vi "sv_Extract Indices from RPM Curve.vi"(2 "rpm segment":T1={"from [rpm]"=2000.0, "to [rpm]"=4000.0, "rpm increment [rpm]"=100.0} {"rpm increment [rpm]" min=1.0 format="%.2f"; "to [rpm]" format="%.2f"; "from [rpm]" format="%.2f"}, 3 "rpm vs. indices":cluster{"indices":dbl[], "speed [rpm]":dbl[]} {"speed [rpm]" format="%.2f"; "indices" format="%.2f"}) -> (0 "rpm0 and delta rpm [rpm]":cluster{"rpm0":dbl, "delta rpm":dbl} {"delta rpm" format="%.2f"; "rpm0" format="%.2f"}, 1 "indices":i32[](array[numeric]))   [LabVIEW 2017]
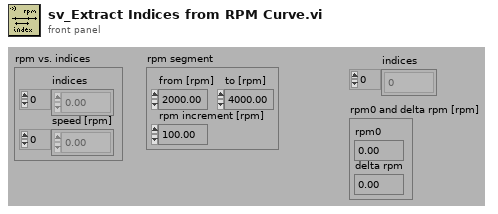
[diagram p1: front panel]
types:
  T1 = cluster{"from [rpm]":dbl, "to [rpm]":dbl, "rpm increment [rpm]":dbl}
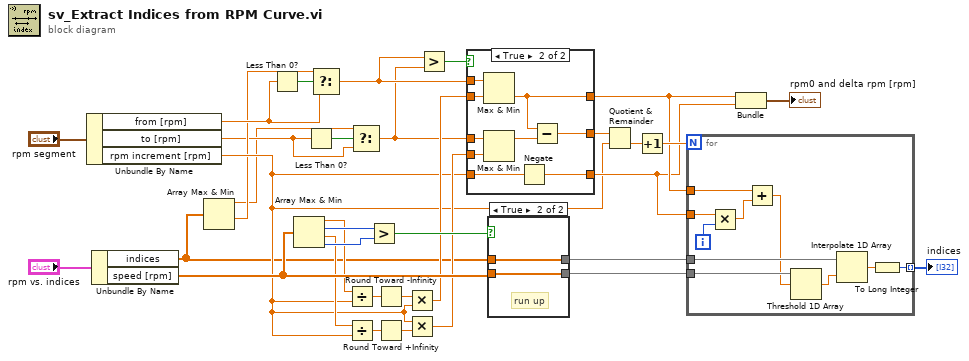
[diagram p0: block diagram]
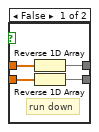
[diagram p2: hidden frame]
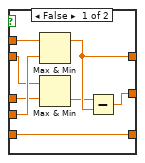
[diagram p3: hidden frame]
diagram:
  n1 = Unbundle By Name("rpm segment") -> ("from [rpm]"=w8:dbl, "to [rpm]"=w3:dbl, "rpm increment [rpm]"=w11:dbl)
  n2 = Unbundle By Name("rpm vs. indices") -> ("indices"=w6:dbl[], "speed [rpm]"=w28:dbl[])
  n3 = Array Max & Min(array=w6) -> (max value=w1:dbl, min value=w5:dbl)  [unwired: 2 out]
  n4 = Less Than 0?(x=w8) -> (x < 0?=w9:bool)
  n5 = Array Max & Min(array=w28) -> (max value=w23:dbl, max index (indices)=w27:i32, min value=w20:dbl, min index (indices)=w26:i32)
  n6 = Less Than 0?(x=w3) -> (x < 0?=w4:bool)
  n7 = Select(t=w5, s=w9, f=w8) -> (s? t:f=w7:dbl)
  n8 = Divide(x=w23, y=w11) -> (x/y=w22:dbl)
  n9 = Divide(x=w20, y=w11) -> (x/y=w19:dbl)
  n10 = Select(t=w1, s=w4, f=w3) -> (s? t:f=w2:dbl)
  n11 = Greater?(x=w27, y=w26) -> (0:w25:bool)
  n12 = Round Toward -Infinity(1:w22) -> (0:w21:dbl)
  n13 = Round Toward +Infinity(x=w19) -> (ceil(x): smallest int >= x=w18:dbl)
  n14 = Multiply(x=w21, y=w11) -> (x*y=w16:dbl)
  n15 = Multiply(x=w11, y=w18) -> (x*y=w17:dbl)
  n16 = Greater?(x=w7, y=w2) -> (0:w24:bool)
  n17 = case shown="True" w24 {
    tunnel: w11 -> [w42 w51]
    tunnel: [w42 w50] -> w13
    tunnel: [w37 w49] -> w30
    tunnel: w2 -> [w39 w48]
    tunnel: w17 -> [w40 w47]
    tunnel: w16 -> [w38 w46]
    tunnel: w7 -> [w41 w45]
    tunnel: [w36 w43] -> w14
    frame False {
      n18 = Max & Min(x=w41, y=w40) -> (max(x,y)=w36:dbl)  [unwired: 1 out]
      n19 = Max & Min(x=w38, y=w39) -> (min(x,y)=w35:dbl)  [unwired: 1 out]
      n20 = Subtract(x=w35, y=w36) -> (x-y=w37:dbl)
    }
    frame True {
      n21 = Max & Min(x=w45, y=w46) -> (min(x,y)=w43:dbl)  [unwired: 1 out]
      n22 = Max & Min(x=w48, y=w47) -> (max(x,y)=w44:dbl)  [unwired: 1 out]
      n23 = Negate(x=w51) -> (-x=w50:dbl)
      n24 = Subtract(x=w43, y=w44) -> (x-y=w49:dbl)
    }
  }
  n25 = case shown="True" w25 {
    tunnel: [w55 w56] -> w33
    tunnel: [w54 w57] -> w32
    tunnel: w6 -> [w53 w57]
    tunnel: w28 -> [w52 w56]
    frame False {
      # "run down"
      n26 = Reverse 1D Array(array=w53) -> (reversed array=w54:dbl[])
      n27 = Reverse 1D Array(array=w52) -> (reversed array=w55:dbl[])
    }
    frame True {
      # "run up"
    }
  }
  n28 = Quotient & Remainder(x=w30, y=w11) -> (floor(x/y)=w31:dbl)  [unwired: 1 out]
  n29 = Increment(x=w31) -> (x+1=w29:dbl)
  n30 = for {
    N: w29 -> [_]
    tunnel: w14 -> [w67]
    tunnel: w13 -> [w66]
    tunnel: w33 -> [w63]
    tunnel: w32 -> [w62]
    tunnel: [w58] -> w15 mode=indexing
    i -> [w65]
    n31 = Multiply(x=w66, y=w65) -> (x*y=w64:dbl)
    n32 = Add(x=w67, y=w64) -> (x+y=w59:dbl)
    n33 = Threshold 1D Array(2:w59, 3:w63) -> (0:w60:dbl)  [unwired: 1 in]
    n34 = Interpolate 1D Array(1:w60, 2:w62) -> (0:w61:dbl)
    n35 = To Long Integer(number=w61) -> (32bit integer=w58:i32)
  }
  "indices" <- w15
  n36 = Bundle(w14, "rpm increment [rpm]"=w13) -> (→"rpm0 and delta rpm [rpm]":cluster{dbl, "rpm increment [rpm]":dbl})  [unwired: 1 in]
